vi "Deep Copy Priv.vi"(0 "Tree Dictionary In":variant, 2 "New Parent ID":string, 7 "Unique ID":string, 11 "error in":errorcluster) -> (4 "Tree Dictionary Out":variant, 8 "ID":string, 15 "error out":errorcluster)   [LabVIEW 2016, in "Tree Manager.lvclass"]
uses:
  Tree Manager.lvclass
  Typedefs/Tree.ctl
  Tree Data/Tree Data.lvclass
  <vilib>/Utility/error.llb/Error Cluster From Error Code.vi
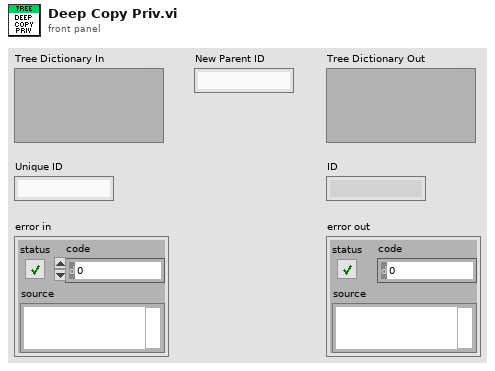
[diagram p1: front panel]
types:
  T1 = typedef "Tree Manager.lvclass/Tree.ctl" = cluster{"Unique ID":string, "Parent ID":string, "Child IDs":string[], "Data":variant, "Name":string}
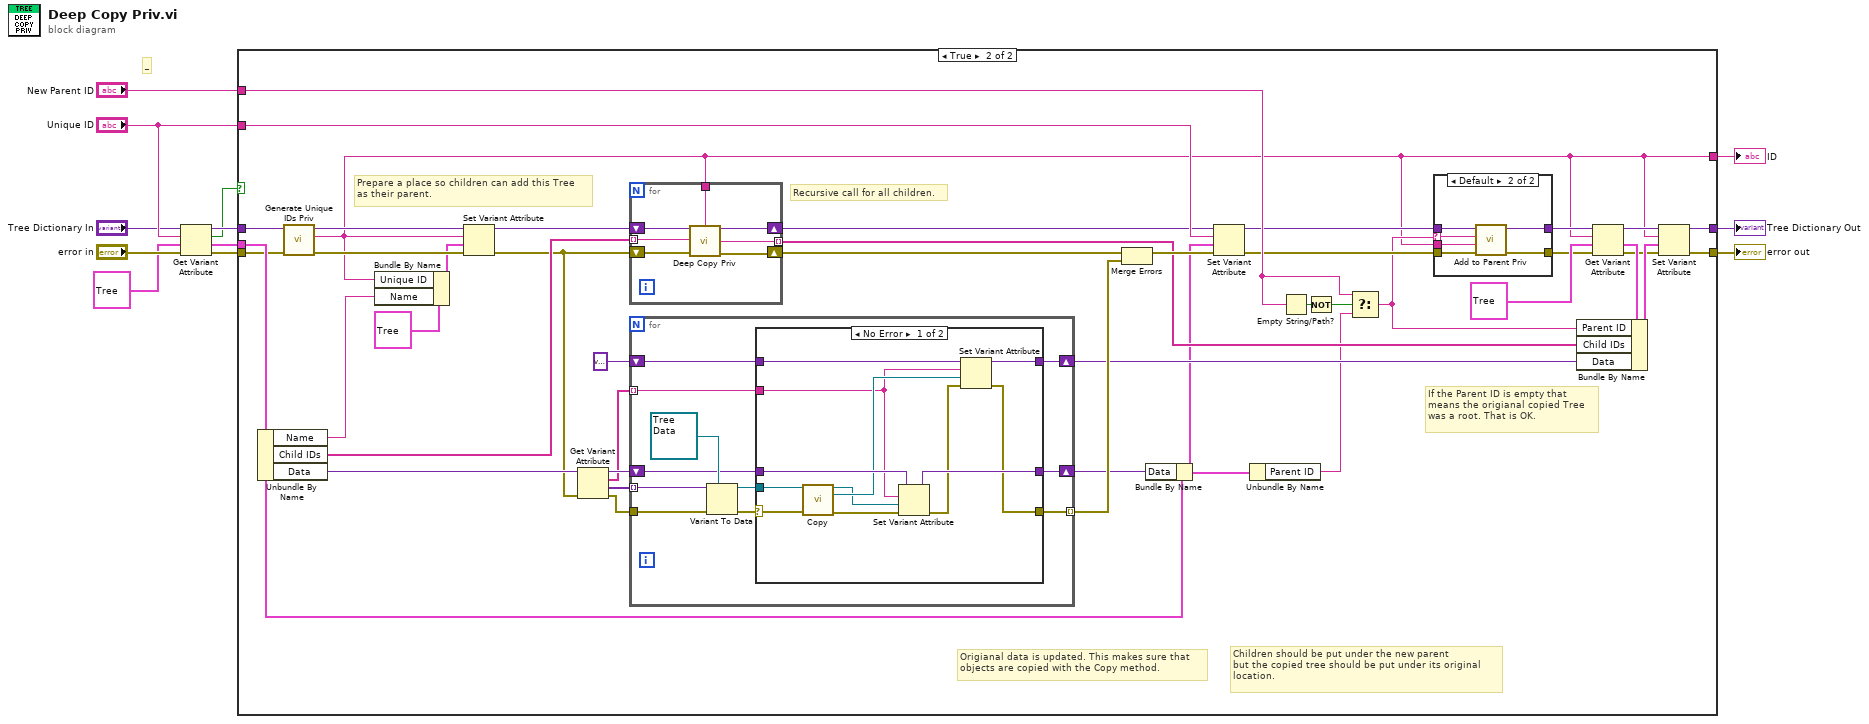
[diagram p0: block diagram]
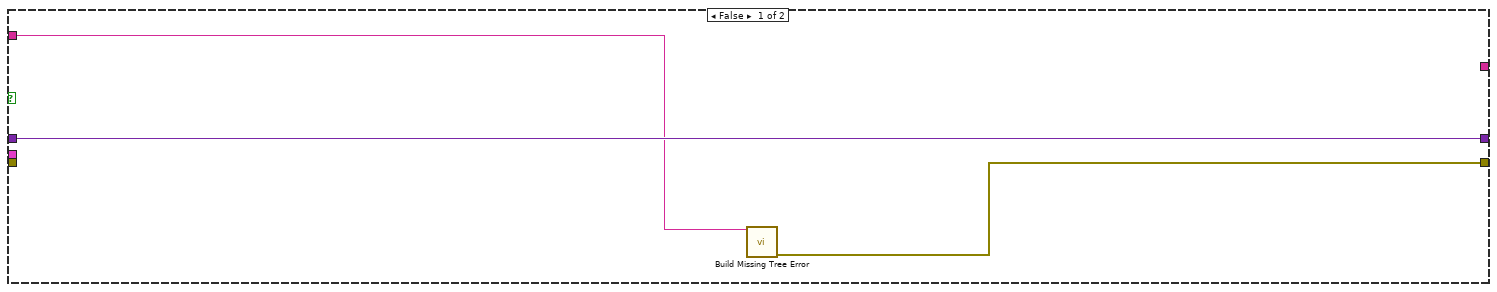
[diagram p2: hidden frame]
diagram:
  # "_"
  n1 = Get Variant Attribute(Variant="Tree Dictionary In", name="Unique ID", default value (empty Variant)=T1 {"Unique ID"="", "Parent ID"="", "Child IDs"=[], "Data"=variant, "Name"=""} ("Cluster of class private data"), error in="error in") -> (duplicate Variant=w6:variant, found=w4:bool, value=w5:T1, error out=w7:errorcluster)
  n2 = case shown="True" w4 {
    tunnel: w5 -> [_ w50]
    tunnel: w6 -> [w15 w41]
    tunnel: w7 -> [_ w40]
    tunnel: [w13 w18] -> w10
    tunnel: [w15 w19] -> w9
    tunnel: "Unique ID" -> [w14 w47]
    tunnel: [_ w16] -> w3
    tunnel: "New Parent ID" -> [_ w37]
    frame False {
      n3 = call "Build Missing Tree Error.vi"("Unique ID"=w14) -> ("Error Out"=w13:errorcluster)  [unwired: 14 in]
    }
    frame True {
      # "Prepare a place so children can add this Tree\nas their parent."
      # "If the Parent ID is empty that\nmeans the origianal copied Tree\nwas a root. That is OK."
      # "Children should be put under the new parent\nbut the copied tree should be put under its original\nlocation."
      # "Origianal data is updated. This makes sure that\nobjects are copied with the Copy method."
      # "Recursive call for all children."
      n4 = Unbundle By Name(w50) -> ("Name"=w17:string, "Child IDs"=w45:string[], "Data"=w58:variant)
      n5 = call "Generate Unique IDs Priv.vi"("Error In"=w40, "Tree Dictionary"=w41) -> ("Error Out"=w34:errorcluster, "First ID"=w16:string, "Tree Dictionary Out"=w35:variant)  [unwired: 6 in, 1 out]
      n6 = Bundle By Name(cluster=T1 {"Unique ID"="", "Parent ID"="", "Child IDs"=[], "Data"=variant, "Name"=""} ("output cluster"), "Unique ID"=w16, "Name"=w17) -> (w32:T1)
      n7 = Set Variant Attribute(Variant=w35, name=w16, value=w32, error in=w34) -> (Variant out=w31:variant, error out=w30:errorcluster)  [unwired: 1 out]
      n8 = Get Variant Attribute(Variant=w58, error in=w30) -> (duplicate Variant=w56:variant, names=w53:string[], values=w57:variant[], error out=w55:errorcluster)  [unwired: 2 in]
      n9 = for {
        shift-right: [w64] -> w42
        shift-left: w31 -> [w65]
        shift-right: [w62] -> w43
        shift-left: w30 -> [w63]
        tunnel: w45 -> [w61] mode=indexing
        tunnel: [w60] -> w44 mode=indexing
        tunnel: w16 -> [w59]
        n10 = call "Deep Copy Priv.vi"("Tree Dictionary In"=w65, "New Parent ID"=w59, "Unique ID"=w61, "error in"=w63) -> ("Tree Dictionary Out"=w64:variant, "ID"=w60:string, "error out"=w62:errorcluster)  [unwired: 9 in]
      }
      n11 = for {
        tunnel: w57 -> [w76] mode=indexing
        shift-right: [w68] -> w49
        shift-left: w56 -> [w71]
        shift-right: [w69] -> w48
        shift-left: variant ("duplicate variant") -> [w70]
        tunnel: w53 -> [w67] mode=indexing
        tunnel: w55 -> [w72]
        tunnel: [w66] -> w52 mode=indexing
        n12 = Variant To Data(error in=w72, type=refnum<class "Tree Data.lvclass"> refnum ("Tree Data.lvclass"), Variant=w76) -> (data=w73:refnum<class "Tree Data.lvclass">, error out=w74:errorcluster)
        n13 = case shown="No Error" w74 {
          selector: w74 -> [w80 _]
          tunnel: w73 -> [w88 _]
          tunnel: w71 -> [w87 w89]
          tunnel: w70 -> [w86 w90]
          tunnel: [w85 w90] -> w69
          tunnel: [w84 w89] -> w68
          tunnel: w67 -> [w81 _]
          tunnel: [w77 _] -> w66
          frame No Error {
            n14 = call-dynamic "Copy.vi"("Tree Data"=w88, "Error In"=w80) -> ("Original"=w82:refnum<class "Tree Data.lvclass">, "Copy"=w83:refnum<class "Tree Data.lvclass">, "Error Out"=w79:errorcluster)  [unwired: 11 in]
            n15 = Set Variant Attribute(Variant=w87, name=w81, value=w82, error in=w79) -> (Variant out=w84:variant, error out=w78:errorcluster)  [unwired: 1 out]
            n16 = Set Variant Attribute(Variant=w86, name=w81, value=w83, error in=w78) -> (Variant out=w85:variant, error out=w77:errorcluster)  [unwired: 1 out]
          }
          frame Error {
          }
        }
      }
      n17 = Merge Errors(w43, w52) -> (w51:errorcluster)
      n18 = Bundle By Name(cluster=w50, "Data"=w49) -> (w25:T1)
      n19 = Set Variant Attribute(Variant=w42, name=w47, value=w25, error in=w51) -> (Variant out=w24:variant, error out=w23:errorcluster)  [unwired: 1 out]
      n20 = Unbundle By Name(w25) -> ("Parent ID"=w36:string)
      n21 = Empty String/Path?(string/path=w37) -> (empty?=w39:bool)
      n22 = Not(x=w39) -> (.not. x?=w38:bool)
      n23 = Select(t=w37, s=w38, f=w36) -> (s? t:f=w22:string)
      n24 = case shown="Default" w22 {
        selector: w22 -> [_ w93]
        tunnel: w24 -> [w92 w98]
        tunnel: w23 -> [w91 w97]
        tunnel: [w91 w96] -> w20
        tunnel: [w92 w95] -> w21
        tunnel: w16 -> [_ w94]
        frame "" {
        }
        frame Default {
          n25 = call "Add to Parent Priv.vi"("Error In"=w97, "Unique ID"=w94, "Parent ID"=w93, "Tree Dictionary"=w98) -> ("Error Out"=w96:errorcluster, "Tree Dictionary Out"=w95:variant)  [unwired: 6 in]
        }
      }
      n26 = Get Variant Attribute(Variant=w21, name=w16, default value (empty Variant)=T1 {"Unique ID"="", "Parent ID"="", "Child IDs"=[], "Data"=variant, "Name"=""} ("output cluster"), error in=w20) -> (duplicate Variant=w26:variant, value=w28:T1, error out=w27:errorcluster)  [unwired: 1 out]
      n27 = Bundle By Name(cluster=w28, "Parent ID"=w22, "Child IDs"=w44, "Data"=w48) -> (w46:T1)
      n28 = Set Variant Attribute(Variant=w26, name=w16, value=w46, error in=w27) -> (Variant out=w19:variant, error out=w18:errorcluster)  [unwired: 1 out]
    }
  }
  "error out" <- w10
  "Tree Dictionary Out" <- w9
  "ID" <- w3
